vi "RemoveObstacle.vi"(8 "error in (no error)":errorcluster, 10 "ID to delete":i32, 11 "Obstacle Notifier":refnum<notifier>) -> (0 "error out":errorcluster)   [LabVIEW 2013]
doc: "This VI removes an obstacle with an indicated ID from the notifier array that it was stored in.\n\nEric Schneider, August 2014"
uses:
  Classes/Obstacle/Obstacle.lvclass
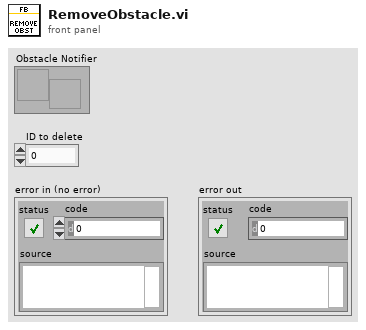
[diagram p1: front panel]
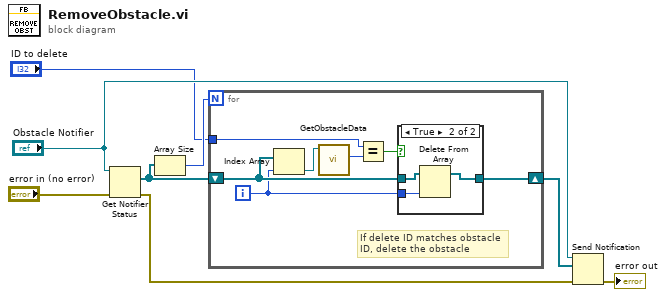
[diagram p0: block diagram]
diagram:
  n1 = Get Notifier Status(notifier="Obstacle Notifier", error in (no error)="error in (no error)") -> (current notification=w4:refnum<class "Obstacle.lvclass">[], error out=w8:errorcluster)  [unwired: 3 out]
  n2 = Array Size(array=w4) -> (size(s)=w3:i32)
  n3 = for {
    N: w3 -> [_]
    tunnel: "ID to delete" -> [w13]
    shift-right: [w11] -> w5
    shift-left: w4 -> [w15]
    i -> [w12]
    # "If delete ID matches obstacle ID, delete the obstacle"
    n4 = Index Array(array=w15, index=w12) -> (element=w10:refnum<class "Obstacle.lvclass">)
    n5 = call "GetObstacleData.vi"("Obstacle.lvclass"=w10) -> ("ID#"=w9:i32)  [unwired: 7 in, 3 out]
    n6 = Equal?(x=w13, y=w9) -> (x = y?=w14:bool)
    n7 = case shown="True" w14 {
      tunnel: w15 -> [w16 w19]
      tunnel: w12 -> [_ w18]
      tunnel: [w16 w17] -> w11
      frame False {
      }
      frame True {
        n8 = Delete From Array(array=w19, index=w18) -> (array with subset deleted=w17:refnum<class "Obstacle.lvclass">[])  [unwired: 1 in, 1 out]
      }
    }
  }
  n9 = Send Notification(notification=w5, notifier="Obstacle Notifier", error in (no error)=w8) -> (error out=→"error out":errorcluster)  [unwired: 1 out]
